vi "genTabx.vi"(11 "Cluster":T1) -> (3 "Ramp Pattern":dbl[](array[numeric]))   [LabVIEW 2020]
uses:
  <vilib>/Analysis/1siggen.llb/Ramp Pattern by Samples.vi
  <vilib>/Analysis/NI_AALBase.lvlib
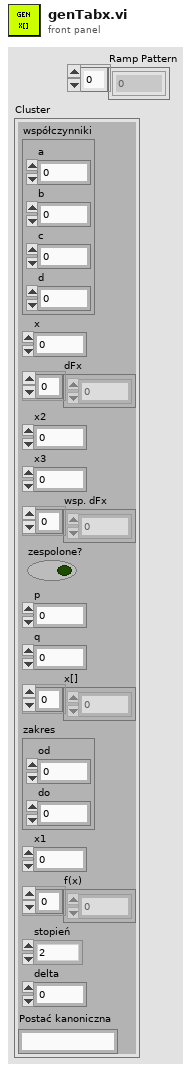
[diagram p1: front panel]
types:
  T1 = cluster{"współczynniki":cluster{"a":dbl, "b":dbl, "c":dbl, "d":dbl}, "x":dbl, "dFx":dbl[], "x2":cdb, "x3":cdb, "wsp. dFx":dbl[], "zespolone?":bool, "p":dbl, "q":dbl, "x[]":dbl[], "zakres":cluster{"od":dbl, "do":dbl}, "x1":cdb, "f(x)":dbl[], "stopień":enum16{"2", "3", "1"}, "delta":i16, "Postać kanoniczna":string}
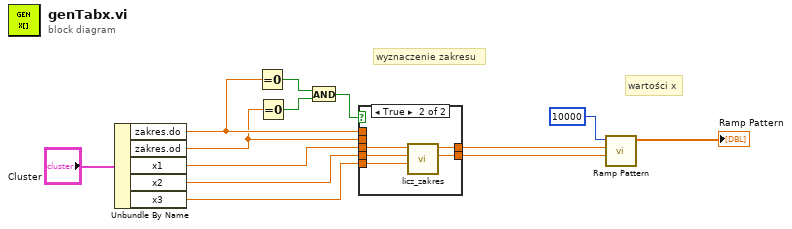
[diagram p0: block diagram]
diagram:
  # "wyznaczenie zakresu"
  # "wartości x"
  n1 = Unbundle By Name("Cluster") -> ("zakres.do"=w5:dbl, "zakres.od"=w4:dbl, "x1"=w3:cdb, "x2"=w2:cdb, "x3"=w1:cdb)
  n2 = Equal To 0?(x=w5) -> (x = 0?=w10:bool)
  n3 = Equal To 0?(x=w4) -> (x = 0?=w11:bool)
  n4 = And(x=w10, y=w11) -> (x .and. y?=w12:bool)
  n5 = case shown="True" w12 {
    tunnel: [w14 w20] -> w7
    tunnel: [w15 w19] -> w8
    tunnel: w3 -> [_ w18]
    tunnel: w2 -> [_ w17]
    tunnel: w1 -> [_ w16]
    tunnel: w4 -> [w15 _]
    tunnel: w5 -> [w14 _]
    frame False {
    }
    frame True {
      n6 = call "licz_zakres.vi"("x3"=w16, "x2"=w17, "x1"=w18) -> ("lewy zakres"=w19:dbl, "prawy zakres"=w20:dbl)  [unwired: 7 in]
    }
  }
  n7 = call-poly <vilib>:"Ramp Pattern.vi"("start"=w8, "end"=w7, "samples"=10000) -> ("Ramp Pattern"=→"Ramp Pattern":dbl[])  [unwired: 7 in, 1 out]
